vi "Start HTTP.vi"(8 "error in (no error)":errorcluster, 11 "Vecto in":refnum<class "Vecto.lvclass">) -> (0 "error out":errorcluster, 3 "Vecto out":refnum<class "Vecto.lvclass">)   [LabVIEW 2020, in "Vecto.lvlib" / "Vecto.lvclass"]
uses:
  Vecto.lvclass
  Vecto.lvclass/Vecto.ctl
  lv-http-server/HTTP Server/Server/Server.lvclass
  Node Config/Node Config.lvclass
  Connection Type.ctl
  Vecto.lvlib
  Connection Info.ctl
  VectoService/VectoInfo.lvclass
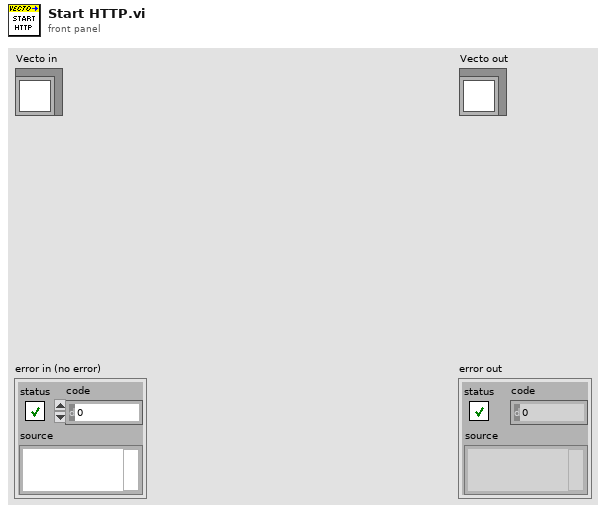
[diagram p1: front panel]
types:
  T1 = typedef "Vecto.lvlib/Connection Type.ctl" = enum16{"TCP", "Telemetry", "Discovery", "HTTP"}
  T2 = typedef "Vecto.lvlib/Connection Info.ctl" = cluster{"Name":string, "Type":T1, "RXCount":i32, "TXCount":i32, "Connected":bool, "RemoteIP":u32, "RemotePort":u16, "LocalPort":u16, "Node ID":u32}
  T3 = typedef "VectoConfig.lvlib/HTTP Server Info.ctl" = cluster{"HTTP Port":u16, "Debug":bool}
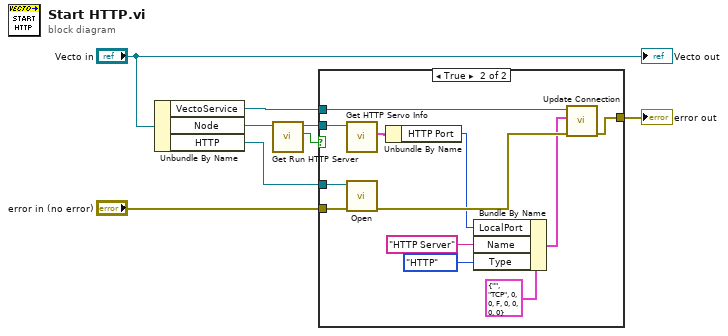
[diagram p0: block diagram]
diagram:
  n1 = Unbundle By Name("Vecto in") -> ("VectoService"=w7:refnum<class "VectoInfo.lvclass">, "Node"=w4:refnum<class "Node Config.lvclass">, "HTTP"=w1:refnum<class "Server.lvclass">)
  n2 = call "Get Run HTTP Server.vi"("Node Config in"=w4) -> ("Run HTTP Server"=w2:bool, "Node Config out"=w3:refnum<class "Node Config.lvclass">)  [unwired: 8 in, 1 out]
  n3 = case shown="True" w2 {
    tunnel: "error in (no error)" -> [w9 w20]
    tunnel: w7 -> [_ w15]
    tunnel: [w9 w10] -> w6
    tunnel: w3 -> [_ w12]
    tunnel: w1 -> [_ w11]
    frame False {
    }
    frame True {
      n4 = call "Get HTTP Servo Info.vi"("Node in"=w12) -> ("HTTP Server Info"=w14:T3)  [unwired: 8 in, 2 out]
      n5 = call "Open.vi"("error in (no error)"=w20, "Server in"=w11) -> ("error out"=w21:errorcluster)  [unwired: 8 in, 1 out]
      n6 = Unbundle By Name(w14) -> ("HTTP Port"=w13:u16)
      n7 = Bundle By Name(cluster=T2 {"Name"="", "Type"=enum."TCP", "RXCount"=0, "TXCount"=0, "Connected"=FALSE, "RemoteIP"=0, "RemotePort"=0, "LocalPort"=0, "Node ID"=0} ("Connection Info"), "LocalPort"=w13, "Name"="HTTP Server", "Type"=Connection_Type."HTTP") -> (w16:T2)
      n8 = call "Update Connection.vi"("error in (no error)"=w21, "Connection Info"=w16, "VectoService in"=w15) -> ("error out"=w10:errorcluster)  [unwired: 7 in, 1 out]
    }
  }
  "error out" <- w6
  "Vecto out" <- "Vecto in"
